vi "Chrg_Dschrg_PTB.vi"(0 "Data Task in":refnum<k21>, 1 "data task error in":errorcluster, 2 "#DAQ outputs (1-13)":i32, 4 "PS VISA in 2":refnum<visa-resource-name>, 5 "PS error in 2":errorcluster, 6 "CyclePath 2":path=path "C:/Users/ga11/Desktop/VI/results/3PtestCharge.lvm" caption="Filename", 8 "Charge/discharge 2":enum8{"Charge", "Discharge"}(ring), 9 "Charge/Discharge Voltage Setpoint  2":dbl format="%#.6g", 10 "CC or CCCV 2":enum16{"CC", "CCCV"}(ring), 11 "Current Setpoint 2":dbl format="%#.6g", 13 "Current Cutoff 2":dbl) -> (14 "data task out":refnum<k21>, 15 "data task error out":errorcluster, 18 "PS VISA out":refnum<visa-resource-name>, 19 "PS error out 2":errorcluster)   [LabVIEW 2020]
uses:
  Parallel-Current-Analysis-Platform-PCAP/parallel_testbed/IT-M3400-LV/IT-M3400/IT-M3400.lvlib
panel:
  out "Read Voltage(V)":dbl format="%.2g"
  out "Read Current(A)":dbl format="%.2g"
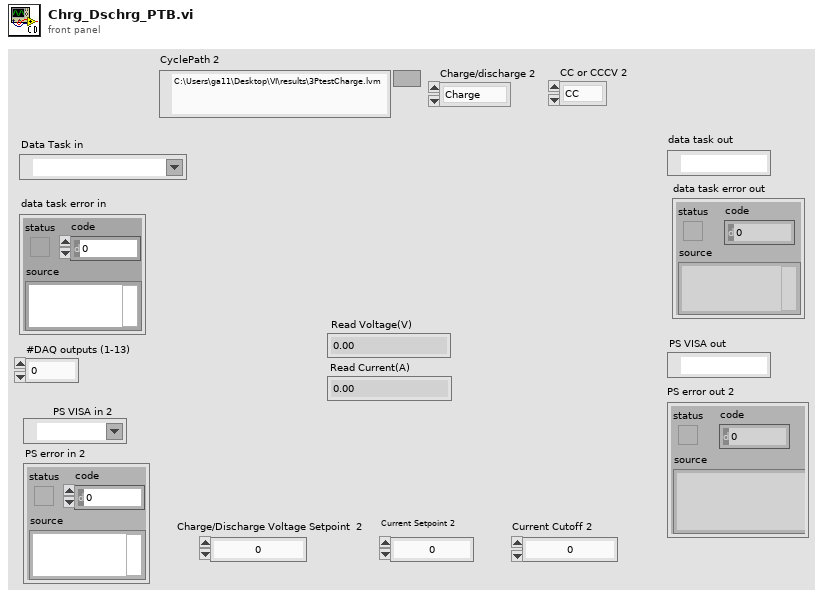
[diagram p1: front panel]
types:
  T1 = enum16{"\"30Q\"", "\"40T\"", "\"2P30Q\"", "\"3P30Q\"", "\"Nissan Leaf\""}
  T2 = cluster{"Baud Rate":u32, "Parity":u16, "Data Bits":u16, "Stop Bits":u16, "Flow Control":u16}
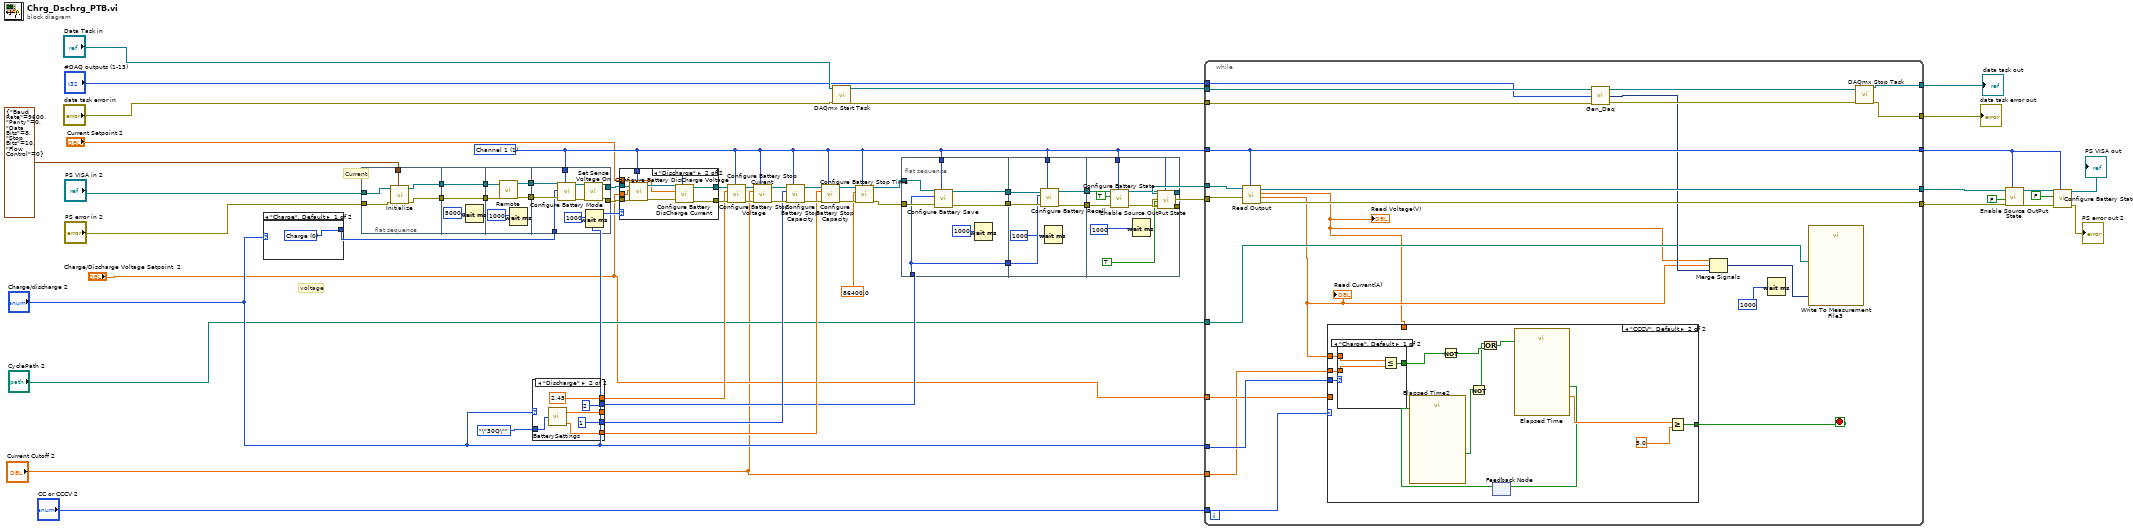
[diagram p0: block diagram]
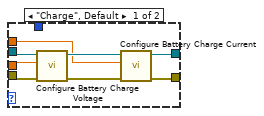
[diagram p2: hidden frame]
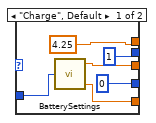
[diagram p3: hidden frame]
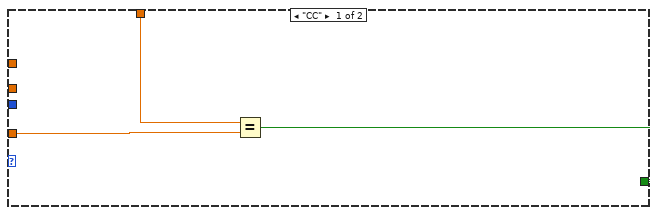
[diagram p4: hidden frame]
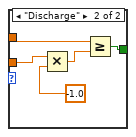
[diagram p5: hidden frame]
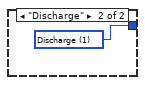
[diagram p6: hidden frame]
diagram:
  w21 = 1 items=["Channel 1"=1, "Channel 2"=2, "Channel 3"=3, "Channel 4"=4, "Channel 5"=5, "Channel 6"=6, "Channel 7"=7, "Channel 8"=8, "Channel 8"=9, "Channel 10"=10, "Channel 11"=11, "Channel 12"=12, "Channel 13"=13, "Channel 14"=14, "Channel 15"=15, "Channel 16"=16] ("Channel")
  # "voltage"
  # "Current"
  n1 = case shown="\"Charge\", Default" "Charge/discharge 2" {
    tunnel: [w61 w62] -> w29
    frame "Charge", Default {
      w61 = u8 0 items=["Charge", "Discharge"] ("Battery Mode")
    }
    frame "Discharge" {
      w62 = u8 1 items=["Charge", "Discharge"] ("Battery Mode")
    }
  }
  n2 = flat-sequence {
    tunnel: [w63] -> w55
    tunnel: [w64] -> w54
    tunnel: T2 {"Baud Rate"=9600, "Parity"=0, "Data Bits"=8, "Stop Bits"=10, "Flow Control"=0} ("Serial Configuration") -> [w67]
    tunnel: "PS error in 2" -> [w66]
    tunnel: "PS VISA in 2" -> [w65]
    tunnel: w55 -> [w70]
    tunnel: [w70] -> w53
    tunnel: w54 -> [w69]
    tunnel: [w69] -> w52
    tunnel: [w75] -> w51
    tunnel: [w74] -> w50
    tunnel: w53 -> [w73]
    tunnel: w52 -> [w72]
    tunnel: w51 -> [w81]
    tunnel: w50 -> [w83]
    tunnel: w21 -> [w84]
    tunnel: w29 -> [w82]
    tunnel: [w77] -> w18
    tunnel: [w76] -> w17
    frame #0 {
      n3 = call "Initialize.vi"("Serial Configuration"=w67, "error in"=w66, "VISA resource name"=w65) -> ("error out"=w64:errorcluster, "VISA resource name out"=w63:refnum<visa-resource-name>)  [unwired: 7 in]
    }
    frame #1 {
      n4 = Wait (ms)(milliseconds to wait=5000) -> ()  [unwired: 1 out]
    }
    frame #2 {
      n5 = call "Remote.vi"("error in"=w72, "VISA resource name"=w73) -> ("error out"=w74:errorcluster, "VISA resource name out"=w75:refnum<visa-resource-name>)  [unwired: 8 in]
      n6 = Wait (ms)(milliseconds to wait=1000) -> ()  [unwired: 1 out]
    }
    frame #3 {
      n7 = call "Configure Battery Mode.vi"("Channel"=w84, "error in"=w83, "Battery Mode"=w82, "VISA resource name"=w81) -> ("error out"=w78:errorcluster, "VISA resource name out"=w79:refnum<visa-resource-name>)  [unwired: 6 in]
      n8 = call "Set Sense Voltage On.vi"("error in"=w78, "VISA resource name"=w79) -> ("error out"=w77:errorcluster, "VISA resource name out"=w76:refnum<visa-resource-name>)  [unwired: 8 in]
      n9 = Wait (ms)(milliseconds to wait=1000) -> ()  [unwired: 1 out]
    }
  }
  n10 = case shown="\"Discharge\"" "Charge/discharge 2" {
    tunnel: T1."\"30Q\"" ("Battery Type") -> [w90 w96]
    tunnel: [w89 w94] -> _
    tunnel: [u8 0 ("File") u8 1 ("File")] -> w23
    tunnel: [u8 1 ("File") u8 2 ("File")] -> w20
    tunnel: [w86 w92] -> w22
    tunnel: [4.25 2.45] -> w19
    frame "Charge", Default {
      n11 = call "BatterySettings.vi"("Battery Type"=w90) -> ("RatedCapacity (Ah)"=w86:dbl, "Max Voltage (V)"=w89:dbl)  [unwired: 2 in, 1 out]
    }
    frame "Discharge" {
      n12 = call "BatterySettings.vi"("Battery Type"=w96) -> ("RatedCapacity (Ah)"=w92:dbl, "Min Voltage (V)"=w94:dbl)  [unwired: 2 in, 1 out]
    }
  }
  n13 = case shown="\"Discharge\"" "Charge/discharge 2" {
    tunnel: w17 -> [w104 w113]
    tunnel: w18 -> [w103 w112]
    tunnel: [w98 w109] -> w39
    tunnel: [w97 w108] -> w38
    tunnel: w21 -> [_ w107]
    tunnel: "Charge/Discharge Voltage Setpoint  2" -> [w100 w106]
    tunnel: "Current Setpoint 2" -> [w99 w105]
    frame "Charge", Default {
      n14 = call "Configure Battery Charge Voltage.vi"("error in"=w103, "Charge Voltage(V)"=w100, "VISA resource name"=w104) -> ("error out"=w101:errorcluster, "VISA resource name out"=w102:refnum<visa-resource-name>)  [unwired: 6 in]
      n15 = call "Configure Battery Charge Current.vi"("error in"=w101, "Charge Current(A)"=w99, "VISA resource name"=w102) -> ("error out"=w97:errorcluster, "VISA resource name out"=w98:refnum<visa-resource-name>)  [unwired: 7 in]
    }
    frame "Discharge" {
      n16 = call "Configure Battery DisCharge Voltage.vi"("Channel"=w107, "error in"=w112, "Discharge Voltage(V)"=w106, "VISA resource name"=w113) -> ("error out"=w110:errorcluster, "VISA resource name out"=w111:refnum<visa-resource-name>)  [unwired: 6 in]
      n17 = call "Configure Battery DisCharge Current.vi"("Channel"=w107, "error in"=w110, "Discharge Current(A)"=w105, "VISA resource name"=w111) -> ("error out"=w108:errorcluster, "VISA resource name out"=w109:refnum<visa-resource-name>)  [unwired: 6 in]
    }
  }
  n18 = call "Configure Battery Stop Voltage.vi"("Channel"=w21, "error in"=w38, "Stop Voltage(V)"=w19, "VISA resource name"=w39) -> ("error out"=w46:errorcluster, "VISA resource name out"=w47:refnum<visa-resource-name>)  [unwired: 6 in]
  n19 = call "Configure Battery Stop Current.vi"("Channel"=w21, "error in"=w46, "Stop Current(A)"="Current Cutoff 2", "VISA resource name"=w47) -> ("error out"=w25:errorcluster, "VISA resource name out"=w27:refnum<visa-resource-name>)  [unwired: 6 in]
  n20 = call "Configure Battery Stop Capacity.vi"("Channel"=w21, "error in"=w25, "Stop Capacity(Ah)"=w23, "VISA resource name"=w27) -> ("error out"=w24:errorcluster, "VISA resource name out"=w26:refnum<visa-resource-name>)  [unwired: 6 in]
  n21 = call "Configure Battery Stop Capacity.vi"("Channel"=w21, "error in"=w24, "Stop Capacity(Ah)"=w22, "VISA resource name"=w26) -> ("error out"=w44:errorcluster, "VISA resource name out"=w45:refnum<visa-resource-name>)  [unwired: 6 in]
  n22 = call <vilib>:"DAQmx Start Task.vi"("task/channels in"="Data Task in", "error in"="data task error in") -> ("task out"=w13:refnum<k21>, "error out"=w14:errorcluster)  [unwired: 12 in]
  n23 = call "Configure Battery Stop Time.vi"("Channel"=w21, "error in"=w44, "Stop Time(S)"=86400.0, "VISA resource name"=w45) -> ("error out"=w31:errorcluster, "VISA resource name out"=w30:refnum<visa-resource-name>)  [unwired: 6 in]
  n24 = flat-sequence {
    tunnel: w20 -> [w119]
    tunnel: w21 -> [w114]
    tunnel: [w117] -> w60
    tunnel: [w119] -> w59
    tunnel: [w116] -> w58
    tunnel: w31 -> [w120]
    tunnel: w30 -> [w118]
    tunnel: [w123] -> w57
    tunnel: [w124] -> w56
    tunnel: w60 -> [w127]
    tunnel: w59 -> [w126]
    tunnel: w58 -> [w125]
    tunnel: w21 -> [w121]
    tunnel: [w131] -> w37
    tunnel: [w130] -> w36
    tunnel: w21 -> [w129]
    tunnel: w57 -> [w137]
    tunnel: w56 -> [w136]
    frame #0 {
      n25 = call "Configure Battery Save.vi"("Channel"=w114, "error in"=w120, "File"=w119, "VISA resource name"=w118) -> ("error out"=w117:errorcluster, "VISA resource name out"=w116:refnum<visa-resource-name>)  [unwired: 6 in]
      n26 = Wait (ms)(milliseconds to wait=1000) -> ()  [unwired: 1 out]
    }
    frame #1 {
      n27 = call "Configure Battery Recall.vi"("Channel"=w121, "error in"=w127, "File"=w126, "VISA resource name"=w125) -> ("error out"=w124:errorcluster, "VISA resource name out"=w123:refnum<visa-resource-name>)  [unwired: 6 in]
      n28 = Wait (ms)(milliseconds to wait=1000) -> ()  [unwired: 1 out]
    }
    frame #2 {
      n29 = call "Configure Battery State.vi"("Channel"=w129, "error in"=w136, "State"=TRUE, "VISA resource name"=w137) -> ("error out"=w134:errorcluster, "VISA resource name out"=w135:refnum<visa-resource-name>)  [unwired: 6 in]
      n30 = Wait (ms)(milliseconds to wait=1000) -> ()  [unwired: 1 out]
      n31 = call "Enable Source OutPut State.vi"("Channel"=w129, "error in"=w134, "State"=TRUE ("Enable Output|Intput"), "VISA resource name"=w135) -> ("error out"=w130:errorcluster, "VISA resource name out"=w131:refnum<visa-resource-name>)  [unwired: 6 in]
    }
  }
  n32 = while {
    tunnel: [w158] -> w35
    tunnel: [w156] -> w34
    tunnel: w37 -> [w160]
    tunnel: w36 -> [w159]
    tunnel: w21 -> [w157]
    tunnel: [w157] -> w33
    tunnel: "CyclePath 2" -> [w144]
    tunnel: "Charge/discharge 2" -> [w146]
    tunnel: w14 -> [w149]
    tunnel: w13 -> [w148]
    tunnel: "#DAQ outputs (1-13)" -> [w147]
    tunnel: "CC or CCCV 2" -> [w145]
    tunnel: "Charge/Discharge Voltage Setpoint  2" -> [w141]
    tunnel: "Current Cutoff 2" -> [w140]
    tunnel: [w139] -> w2
    tunnel: [w138] -> w1
    stop <- w150 stop-if-true
    n33 = call "Read Output.vi"("Channel"=w157, "error in"=w159, "VISA resource name"=w160) -> ("error out"=w156:errorcluster, "Actual Current Level (A)"=w143:dbl, "Actual Voltage Level (V)"=w142:dbl, "VISA resource name out"=w158:refnum<visa-resource-name>)  [unwired: 5 in]
    "Read Voltage(V)" <- w142
    "Read Current(A)" <- w143
    n34 = case shown="\"CCCV\", Default" w145 {
      tunnel: [w161 w170] -> w150
      tunnel: w140 -> [_ w167]
      tunnel: w142 -> [w163 _]
      tunnel: w141 -> [w162 _]
      tunnel: w146 -> [_ w165]
      tunnel: w143 -> [_ w164]
      frame "CC" {
        n35 = Equal?(x=w163, y=w162) -> (x = y?=w161:bool)
      }
      frame "CCCV", Default {
        n36 = case shown="\"Charge\", Default" w165 {
          tunnel: w167 -> [w178 w183]
          tunnel: w164 -> [w179 w181]
          tunnel: [w177 w180] -> w166
          frame "Charge", Default {
            n37 = Less Or Equal?(x=w179, y=w178) -> (x <= y?=w177:bool)
          }
          frame "Discharge" {
            n38 = Multiply(x=w183, y=-1.0) -> (x*y=w182:dbl)
            n39 = Greater Or Equal?(x=w181, y=w182) -> (x >= y?=w180:bool)
          }
        }
        n40 = Not(x=w166) -> (.not. x?=w176:bool)
        n41 = feedback #1() -> (w168:bool)  [unwired: 1 in]
        n42 = call "Elapsed Time2"("Reset"=w168) -> ("Time has Elapsed"=w175:bool)  [unwired: 11 in, 7 out]
        n43 = Not(x=w175) -> (.not. x?=w174:bool)
        n44 = Or(x=w174, y=w176) -> (x .or. y?=w173:bool)
        n45 = call "Elapsed Time"("Reset"=w173) -> ("Elapsed Time (s)"=w172:dbl, "Time has Elapsed"=w169:bool)  [unwired: 11 in, 6 out]
        n46 = feedback-in #1(w169) -> ()
        n47 = Greater Or Equal?(x=w172, y=5.0) -> (x >= y?=w170:bool)
      }
    }
    n48 = call "Gen_Daq.vi"("error in"=w149, "#DAQ outputs (1-13)"=w147, "task/channels in"=w148) -> ("error out"=w152:errorcluster, "DaQ_output"=w151:dynamicdata, "task out"=w153:refnum<k21>)
    n49 = Merge Signals "Merge Signals"(w142, w143, w151) -> (w155:dynamicdata)
    n50 = Wait (ms)(milliseconds to wait=1000) -> ()  [unwired: 1 out]
    n51 = call "Write To Measurement File3"("Signals"=w155, "Filename"=w144) -> ()  [unwired: 15 in, 3 out]
    n52 = call <vilib>:"DAQmx Stop Task.vi"("task/channels in"=w153, "error in"=w152) -> ("task out"=w139:refnum<k21>, "error out"=w138:errorcluster)  [unwired: 12 in]
  }
  "data task out" <- w2
  "data task error out" <- w1
  n53 = call "Enable Source OutPut State.vi"("Channel"=w33, "error in"=w34, "State"=FALSE, "VISA resource name"=w35) -> ("error out"=w42:errorcluster, "VISA resource name out"=w43:refnum<visa-resource-name>)  [unwired: 6 in]
  n54 = call "Configure Battery State.vi"("Channel"=w33, "error in"=w42, "State"=FALSE, "VISA resource name"=w43) -> ("error out"=→"PS error out 2":errorcluster, "VISA resource name out"=→"PS VISA out":refnum<visa-resource-name>)  [unwired: 6 in]
